vi "Button press check.vi"(11 "Boolean":bool) -> (3 "Boolean 2":bool)   [LabVIEW 2013]
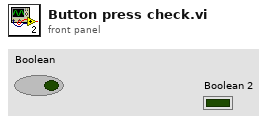
[diagram p1: front panel]
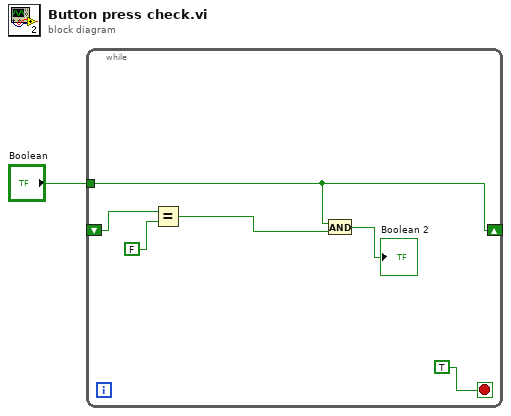
[diagram p0: block diagram]
diagram:
  n1 = while {
    shift-right: [w4] -> _
    shift-left: _ -> [w6]
    tunnel: "Boolean" -> [w4]
    stop <- TRUE stop-if-true
    n2 = Equal?(x=w6, y=FALSE) -> (x = y?=w3:bool)
    n3 = And(x=w4, y=w3) -> (x .and. y?=→"Boolean 2":bool)
  }
